vi "Read NPorts 1Sampe 1D U8.vi"(8 "error in (no error)":errorcluster, 10 "Ports (Banks)":T1[](array[typedef]) items=["DIO1...8"=1, "DIO9...16"=2, "DIO17...24"=3, "DIO25...32"=4], 11 "MicroDAQ.lvlib:Digital Input.lvclass":refnum<class "Digital Input.lvclass">) -> (0 "error out":errorcluster, 2 "data":u8[](array[numeric]) format="%08b", 3 "MicroDAQ.lvlib:Digital Input.lvclass out":refnum<class "Digital Input.lvclass">)   [LabVIEW 2009, in "MicroDAQ.lvlib" / "Digital Input.lvclass"]
doc: "Reads a array of U8 register value from a digital input channel composed of a multiple ports."
uses:
  <instrlib>/MicroDAQ/Channel/Digital Input/Digital Input.lvclass
  <instrlib>/MicroDAQ/Tools/Digital IO channels.ctl
  <instrlib>/MicroDAQ/MicroDAQ.lvlib
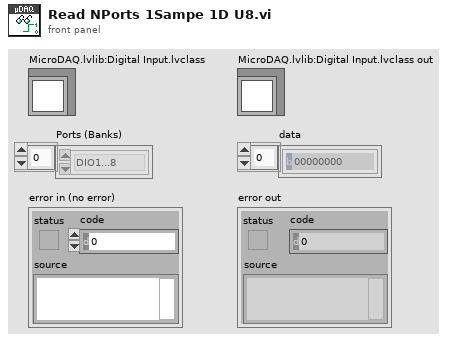
[diagram p1: front panel]
types:
  T1 = typedef "MicroDAQ.lvlib/Digital IO channels.ctl" = u8
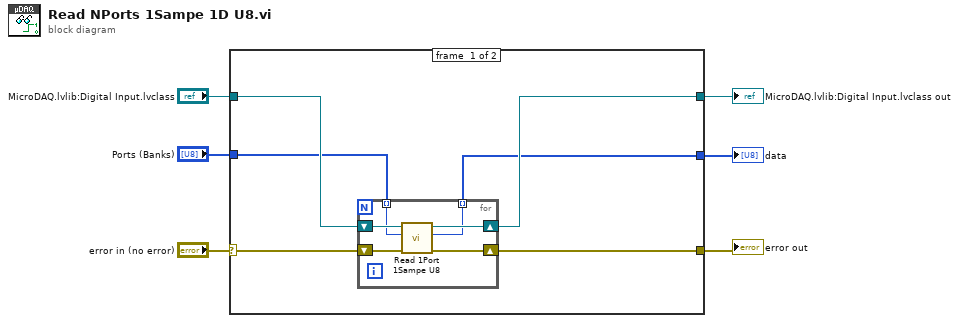
[diagram p0: block diagram]
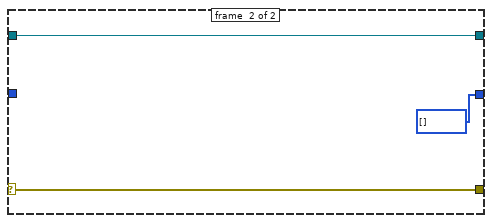
[diagram p2: hidden frame]
diagram:
  n1 = case shown="No Error" "error in (no error)" {
    selector: "error in (no error)" -> [w12 w20]
    tunnel: [w11 w20] -> w5
    tunnel: "MicroDAQ.lvlib:Digital Input.lvclass" -> [w10 w21]
    tunnel: [w9 w21] -> w3
    tunnel: "Ports (Banks)" -> [w8 _]
    tunnel: [w7 u8[] []] -> w1
    frame #0 {
      n2 = for {
        shift-right: [w17] -> w11
        shift-left: w12 -> [w18]
        shift-right: [w15] -> w9
        shift-left: w10 -> [w16]
        tunnel: w8 -> [w14] mode=indexing
        tunnel: [w13] -> w7 mode=indexing
        n3 = call <instrlib>:"Read 1Port 1Sampe U8.vi"("error in (no error)"=w18, "Port (Bank)"=w14, "MicroDAQ.lvlib:Digital Input.lvclass"=w16) -> ("error out"=w17:errorcluster, "data"=w13:u8, "MicroDAQ.lvlib:Digital Input.lvclass out"=w15:refnum<class "Digital Input.lvclass">)  [unwired: 6 in]
      }
    }
    frame #1 {
    }
  }
  "error out" <- w5
  "MicroDAQ.lvlib:Digital Input.lvclass out" <- w3
  "data" <- w1
